vi "Main Page.vi"(8 "error in (no error)":errorcluster, 11 "Node Ptr":T1 format="%.0x") -> (0 "error out":errorcluster)   [LabVIEW 2024, in "Nominal Client System Explorer.lvlib"]
uses:
  Nominal Client System Explorer.lvlib
  <vilib>/NI VeriStand/Custom Device API/Custom Device Item Ref.ctl
  <vilib>/NI VeriStand/Custom Device API/Get Item Property (U16).vi
  <vilib>/NI VeriStand/Custom Device API/Set Item Property (U16).vi
  <vilib>/NI VeriStand/Custom Device API/Custom Device API.lvlib
  Scripting/Nominal Client Scripting.lvlib
  <vilib>/NI VeriStand/Custom Device Tools/Custom Device Utility Library/Custom Device Utility Library.lvlib
panel:
  in  "Remove":bool
  in  "Channels to Stream":i32[](listbox)
  in  "Add Channels":bool
  in  "Datasource Connection Name":string
  in  "Path to API Token file":path caption="A text file containing your API Token only."
  in  "Description":string
  in  "Name":string
  out "Version":string
  in  "General Header":cluster{"Section Name":string}={"Section Name"="Nominal IO VeriStand Client Details"}
  in  "Specific Header":cluster{"Section Name":string}={"Section Name"="Settings"}
  in  "Async Timeout (ms)":u16
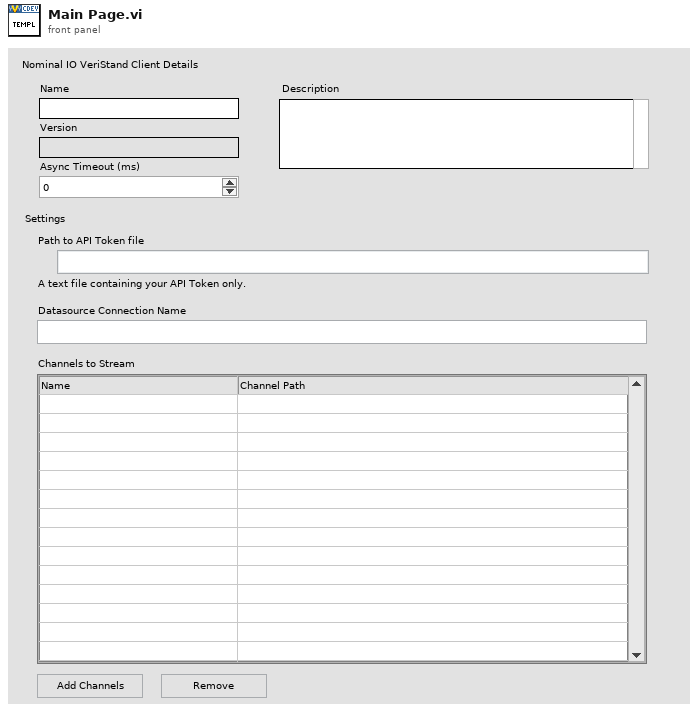
[diagram p1: front panel]
types:
  T1 = typedef "Custom Device API.lvlib/Custom Device Item Ref.ctl" = u64
  T2 = typedef "Custom Device API.lvlib/Custom Device Item Info.ctl" = cluster{"Name":string, "Is Channel":bool, "GUID":string, "Is Waveform":bool}
  T3 = typedef "Custom Device API.lvlib/Custom Device Commands.ctl" = enum16{"Default", "Item renamed", "Shutdown", "Dynamic button pressed"}
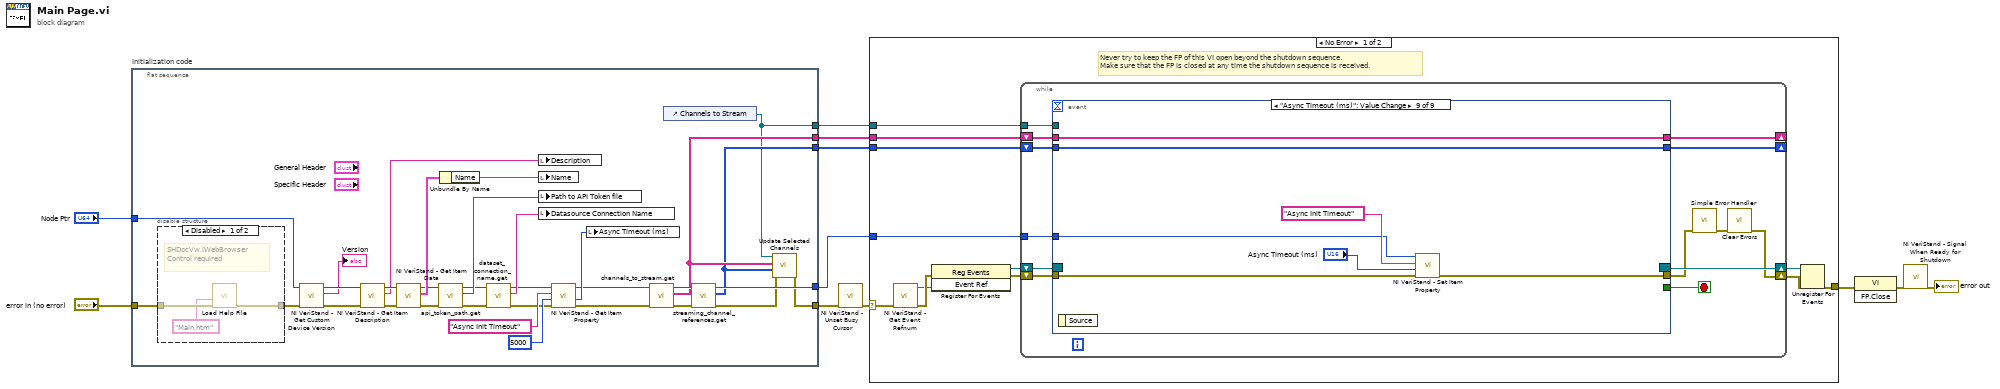
[diagram p0: block diagram]
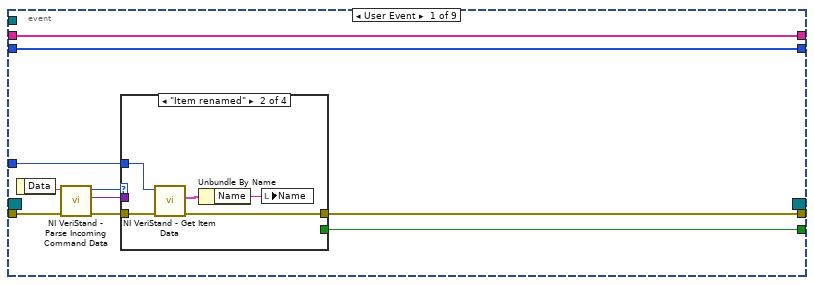
[diagram p2: hidden frame]
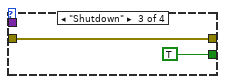
[diagram p4: hidden frame]
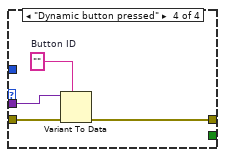
[diagram p5: hidden frame]
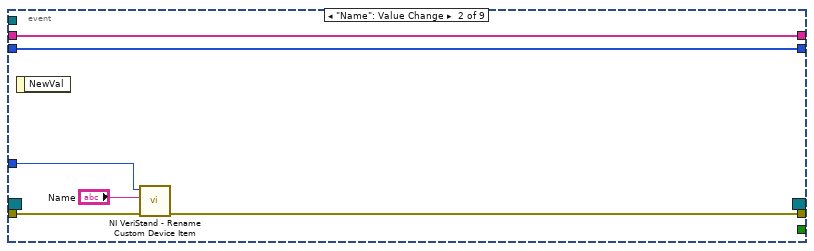
[diagram p6: hidden frame]
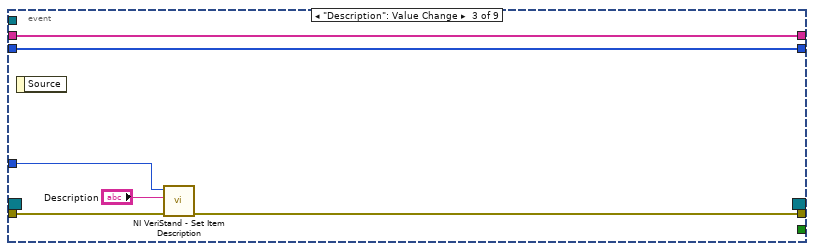
[diagram p7: hidden frame]
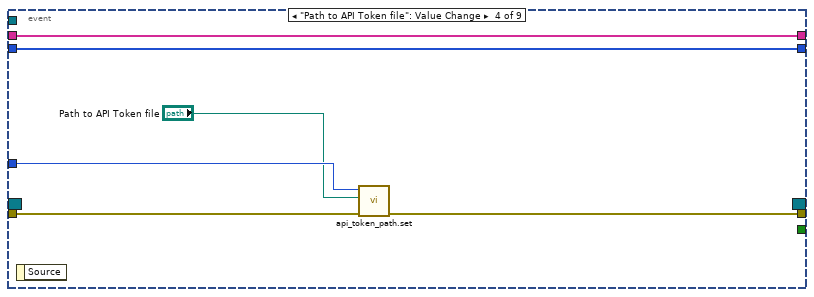
[diagram p8: hidden frame]
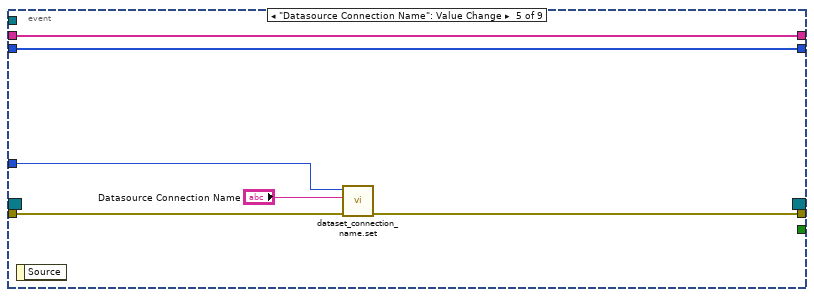
[diagram p9: hidden frame]
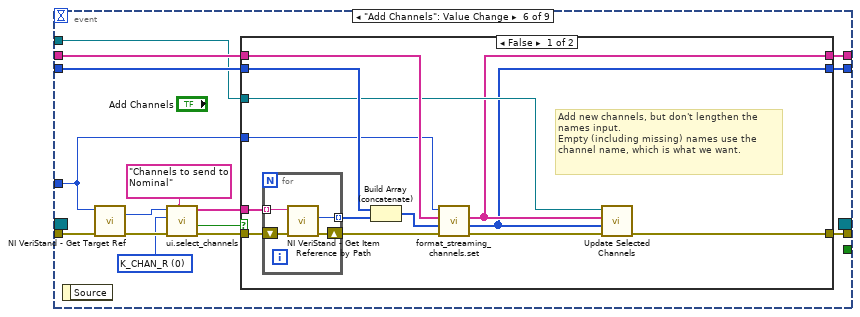
[diagram p10: hidden frame]
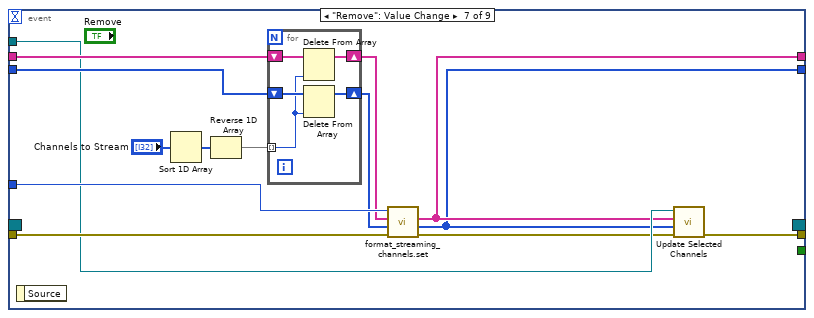
[diagram p12: hidden frame]
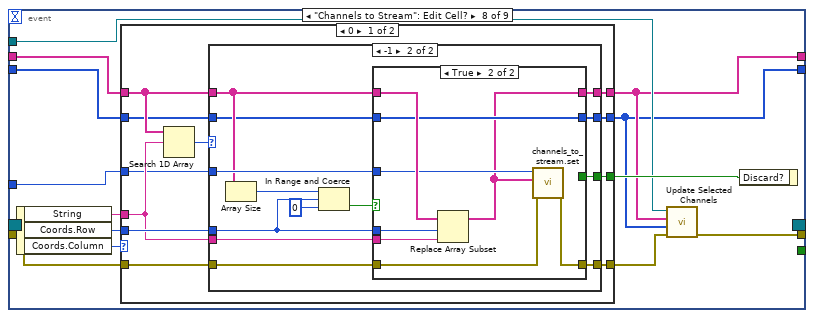
[diagram p13: hidden frame]
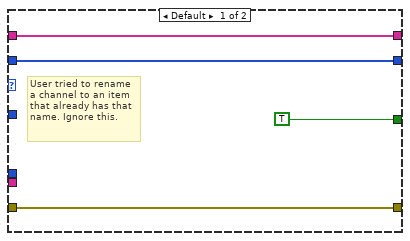
[diagram p14: hidden frame]
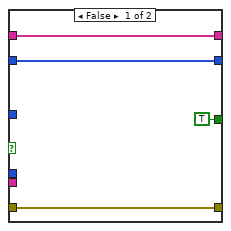
[diagram p15: hidden frame]
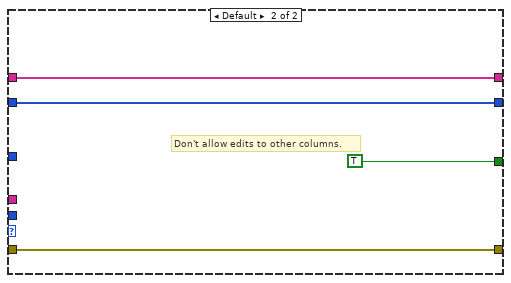
[diagram p16: hidden frame]
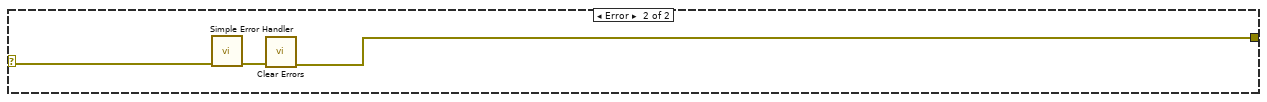
[diagram p17: hidden frame]
diagram:
  n1 = flat-sequence "Initialization code" {
    tunnel: "error in (no error)" -> [w34]
    tunnel: "Node Ptr" -> [w40]
    tunnel: [w20] -> w8
    tunnel: [w26] -> w6
    tunnel: [w22] -> w5
    tunnel: [w23] -> w4
    tunnel: [w19] -> w3
    frame #0 {
      n2 = disable-structure shown="Disabled" {
        disable-tunnel: w34 -> [w46 w47]
        disable-tunnel: [w44 w47] -> w33
        frame Disabled {
          # "SHDocVw.IWebBrowser Control required"
          n3 = call "Load Help File.vi"("error in (no error)"=w46, "HTML File to Load"="Main.htm" ("HTML File")) -> ("error out"=w44:errorcluster)  [unwired: 9 in]
        }
        frame Enabled {
          # "Enable to add help support"
        }
      }
      n4 = call <vilib>:"NI VeriStand - Get Custom Device Version.vi"("error in (no error)"=w33, "Device Ref in"=w40) -> ("error out"=w39:errorcluster, "Value"=→"Version":string, "Device Ref out"=w38:T1)  [unwired: 7 in]
      n5 = call <vilib>:"NI VeriStand - Get Item Description.vi"("error in (no error)"=w39, "Item Ref in"=w38) -> ("error out"=w42:errorcluster, "Description"=w35:string, "Item Ref out"=w43:T1)  [unwired: 7 out]
      n6 = call <vilib>:"NI VeriStand - Get Item Data.vi"("error in (no error)"=w42, "Item Ref in"=w43) -> ("error out"=w31:errorcluster, "Item Info"=w41:T2, "Item Ref out"=w32:T1)  [unwired: 7 out]
      n7 = call "api_token_path.get.vi"("error in (no error)"=w31, "Nominal IO Client in"=w32) -> ("error out"=w28:errorcluster, "API Token file"=w30:path, "Nominal IO Client out"=w29:T1)  [unwired: 6 in, 1 out]
      n8 = Unbundle By Name(w41) -> ("Name"=w36:string)
      n9 = call "dataset_connection_name.get.vi"("error in (no error)"=w28, "Nominal IO Client in"=w29) -> ("error out"=w14:errorcluster, "dataset connection name"=w27:string, "Nominal IO Client out"=w15:T1)  [unwired: 6 in, 1 out]
      n10 = local write "Description"(w35) -> ()
      n11 = local write "Name"(w36) -> ()
      n12 = local write "Path to API Token file"(w30) -> ()
      n13 = local write "Datasource Connection Name"(w27) -> ()
      n14 = call-poly <vilib>:"NI VeriStand - Get Item Property.vi"("error in (no error)"=w14, "Default Value"=u16 5000, "Property Name"="Async Init Timeout", "Item Ref in"=w15) -> ("error out"=w13:errorcluster, "Value"=w18:u16, "Item Ref out"=w12:T1)  [unwired: 4 in, 1 out]
      n15 = local write "Async Timeout (ms)"(w18) -> ()
      n16 = call "channels_to_stream.get.vi"("error in (no error)"=w13, "Nominal IO Client in"=w12) -> ("error out"=w25:errorcluster, "Channels to Stream"=w23:string[], "Nominal IO Client out"=w24:T1)  [unwired: 6 in, 1 out]
      n17 = control-ref of="Channels to Stream"() -> (w19:refnum<vi>)
      n18 = call "streaming_channel_references.get.vi"("error in (no error)"=w25, "Item Ref in"=w24) -> ("error out"=w21:errorcluster, "Streaming Channel Refs"=w22:T1[], "Item Ref out"=w26:T1)  [unwired: 7 in]
      n19 = call "Update Selected Channels.vi"("error in"=w21, "Channel Refs"=w22, "Channel Names"=w23, "Listbox"=w19) -> ("error out"=w20:errorcluster)  [unwired: 7 in]
    }
  }
  n20 = call <vilib>:"NI VeriStand - Unset Busy Cursor.vi"("error in (no error)"=w8) -> ("error out"=w7:errorcluster)  [unwired: 10 out]
  n21 = case shown="No Error" w7 {
    selector: w7 -> [w51 w239]
    tunnel: [w56 w237] -> w11
    tunnel: w6 -> [w52 _]
    tunnel: w5 -> [w50 _]
    tunnel: w4 -> [w49 _]
    tunnel: w3 -> [w48 _]
    frame No Error {
      # "Never try to keep the FP of this VI open beyond the shutdown sequence.\nMake sure that the FP is closed at any time the shutdown sequence is received."
      n22 = call <vilib>:"NI VeriStand - Get Event Refnum.vi"("error in (no error)"=w51) -> ("error out"=w59:errorcluster, "Event Ref"=w55:refnum<user-event>)  [unwired: 9 out]
      n23 = register-events(error in=w59, w55) -> (reference out=w53:refnum<event-registration>, error out=w54:errorcluster)  [unwired: 1 in]
      n24 = while {
        tunnel: w52 -> [w68]
        shift-right: [w65] -> w57
        shift-left: w54 -> [w71]
        shift-right: [w72] -> w58
        shift-left: w53 -> [w70]
        shift-right: [w63] -> _
        shift-left: w50 -> [w64]
        shift-right: [w61] -> _
        shift-left: w49 -> [w62]
        tunnel: w48 -> [w60]
        stop <- w69 stop-if-true
        n25 = event shown="[8] \"Async Timeout (ms)\": Value Change" {
          selector: w70 -> [_ _ _ _ _ _ _ _ _]
          dyn-events: [_ _ _ _ _ _ _ _ _] -> w72
          timeout: _ -> [_ _ _ _ _ _ _ _ _]
          tunnel: w71 -> [w82 w100 w105 w110 w115 w133 w159 w182 w231]
          tunnel: [w73 _ _ _ _ _ _ _ _] -> w69
          tunnel: [w74 w99 w104 w109 w116 w128 w154 w173 w230] -> w67
          tunnel: w68 -> [w75 w98 w106 w112 w117 w127 w162 w183 w232]
          tunnel: w64 -> [w76 w95 w101 w107 w113 w132 w165 w185 w236]
          tunnel: [w76 w95 w101 w107 w113 w131 w156 w175 w236] -> w63
          tunnel: w62 -> [w77 w96 w102 w108 w114 w130 w164 w184 w235]
          tunnel: [w77 w96 w102 w108 w114 w129 w157 w176 w235] -> w61
          tunnel: w60 -> [_ _ _ _ _ w126 w158 w177 _]
          event User Event {
            n26 = event-data() -> ("Data"=w81:string)  [unwired: 1 out]
            n27 = call <vilib>:"NI VeriStand - Parse Incoming Command Data.vi"("error in (no error)"=w82, "Incoming data"=w81) -> ("error out"=w80:errorcluster, "Outgoing data"=w78:variant, "Action"=w79:T3)  [unwired: 7 out]
            n28 = case shown="\"Item renamed\"" w79 {
              tunnel: w80 -> [w83 w88 w89 w94]
              tunnel: [_ _ TRUE _] -> w73
              tunnel: [w83 w85 w89 w91] -> w74
              tunnel: w75 -> [_ w87 _ _]
              tunnel: w78 -> [_ _ _ w93]
              frame "Default", Default {
              }
              frame "Item renamed" {
                n29 = call <vilib>:"NI VeriStand - Get Item Data.vi"("error in (no error)"=w88, "Item Ref in"=w87) -> ("error out"=w85:errorcluster, "Item Info"=w86:T2)  [unwired: 8 out]
                n30 = Unbundle By Name(w86) -> ("Name"=w84:string)
                n31 = local write "Name"(w84) -> ()
              }
              frame "Shutdown" {
              }
              frame "Dynamic button pressed" {
                w92 = ""  # Button ID
                n32 = Variant To Data(error in=w94, type=w92, Variant=w93) -> (error out=w91:errorcluster)  [unwired: 1 out]
              }
            }
          }
          event "Name": Value Change {
            n33 = event-data() -> ()  [unwired: 2 out]
            n34 = call <vilib>:"NI VeriStand - Rename Custom Device Item.vi"("error in (no error)"=w100, "New Name"="Name", "Item Ref in"=w98) -> ("error out"=w99:errorcluster)  [unwired: 1 in, 7 out]
          }
          event "Description": Value Change {
            n35 = event-data() -> ()  [unwired: 2 out]
            n36 = call <vilib>:"NI VeriStand - Set Item Description.vi"("error in (no error)"=w105, "Description"="Description", "Item Ref in"=w106) -> ("error out"=w104:errorcluster)  [unwired: 8 out]
          }
          event "Path to API Token file": Value Change {
            n37 = event-data() -> ()  [unwired: 2 out]
            n38 = call "api_token_path.set.vi"("error in (no error)"=w110, "API Token file"="Path to API Token file", "Nominal IO Client in"=w112) -> ("error out"=w109:errorcluster)  [unwired: 6 in, 2 out]
          }
          event "Datasource Connection Name": Value Change {
            n39 = event-data() -> ()  [unwired: 2 out]
            n40 = call "dataset_connection_name.set.vi"("error in (no error)"=w115, "dataset connection name"="Datasource Connection Name", "Nominal IO Client in"=w117) -> ("error out"=w116:errorcluster)  [unwired: 6 in, 2 out]
          }
          event "Add Channels": Value Change {
            w119 = u8 0 items=["K_CHAN_R", "K_CHAN_W", "K_CHAN_RW", "K_CHAN_VOLT", "K_CHAN_FAULT", "K_ALL", "K_CUSTOM"] ("Filter")
            n41 = event-data() -> ()  [unwired: 2 out]
            n42 = call <vilib>:"NI VeriStand - Get Target Ref.vi"("error in"=w133, "Item Ref in"=w127) -> ("error out"=w124:errorcluster, "Target Ref"=w123:T1)  [unwired: 6 in, 2 out]
            n43 = call "ui.select_channels.vi"("Channel Label"="Channels to send to Nominal", "error in (no error)"=w124, "Filter"=w119, "Start Item Ref"=w123) -> ("error out"=w122:errorcluster, "Canceled"=w121:bool, "Channels"=w120:string[])  [unwired: 5 in]
            n44 = case shown="False" w121 {
              tunnel: w120 -> [w146 _]
              tunnel: w122 -> [w145 w151]
              tunnel: w132 -> [w142 w152]
              tunnel: [w136 w152] -> w131
              tunnel: w130 -> [w141 w153]
              tunnel: [w137 w153] -> w129
              tunnel: [w134 w151] -> w128
              tunnel: w127 -> [w139 _]
              tunnel: w126 -> [w138 _]
              frame False {
                # "Add new channels, but don't lengthen the names input.\nEmpty (including missing) names use the channel name, which is what we want."
                n45 = for {
                  shift-right: [w149] -> w140
                  shift-left: w145 -> [w150]
                  tunnel: w146 -> [w148] mode=indexing
                  tunnel: [w147] -> w144 mode=indexing
                  n46 = call <vilib>:"NI VeriStand - Get Item Reference by Path.vi"("error in (no error)"=w150, "Item Path in"=w148) -> ("error out"=w149:errorcluster, "Item Ref"=w147:T1)  [unwired: 6 in, 2 out]
                }
                n47 = Build Array (concatenate)(w142, w144) -> (w143:T1[])
                n48 = call "format_streaming_channels.set.vi"("error in"=w140, "channels"=w143, "names"=w141, "Nominal IO Client in"=w139) -> ("error out"=w135:errorcluster, "saved channels"=w136:T1[], "saved names"=w137:string[])  [unwired: 4 in, 1 out]
                n49 = call "Update Selected Channels.vi"("error in"=w135, "Channel Refs"=w136, "Channel Names"=w137, "Listbox"=w138) -> ("error out"=w134:errorcluster)  [unwired: 7 in]
              }
              frame True {
              }
            }
          }
          event "Remove": Value Change {
            n50 = event-data() -> ()  [unwired: 2 out]
            n51 = Sort 1D Array(array="Channels to Stream") -> (sorted array=w167:i32[])
            n52 = Reverse 1D Array(array=w167) -> (reversed array=w166:i32[])
            n53 = for {
              shift-right: [w171] -> w160
              shift-left: w165 -> [w172]
              tunnel: w166 -> [w168] mode=indexing
              shift-right: [w169] -> w161
              shift-left: w164 -> [w170]
              n54 = Delete From Array(array=w170, index=w168) -> (array with subset deleted=w169:string[])  [unwired: 1 in, 1 out]
              n55 = Delete From Array(array=w172, index=w168) -> (array with subset deleted=w171:T1[])  [unwired: 1 in, 1 out]
            }
            n56 = call "format_streaming_channels.set.vi"("error in"=w159, "channels"=w160, "names"=w161, "Nominal IO Client in"=w162) -> ("error out"=w155:errorcluster, "saved channels"=w156:T1[], "saved names"=w157:string[])  [unwired: 4 in, 1 out]
            n57 = call "Update Selected Channels.vi"("error in"=w155, "Channel Refs"=w156, "Channel Names"=w157, "Listbox"=w158) -> ("error out"=w154:errorcluster)  [unwired: 7 in]
          }
          event "Channels to Stream": Edit Cell? {
            n58 = event-data() -> ("String"=w178:string, "Coords.Row"=w179:i32, "Coords.Column"=w181:i32)  [unwired: 1 out]
            n59 = case shown="0" w181 {
              tunnel: w185 -> [w191 w228]
              tunnel: w184 -> [w193 w229]
              tunnel: [w194 w229] -> w176
              tunnel: [w192 w228] -> w175
              tunnel: w179 -> [w190 _]
              tunnel: [w195 TRUE] -> w180
              tunnel: w178 -> [w189 _]
              tunnel: w182 -> [w188 w226]
              tunnel: w183 -> [w187 _]
              tunnel: [w186 w226] -> w174
              frame 0 {
                n60 = Search 1D Array(1D array=w193, element=w189) -> (index of element=w196:i32)  [unwired: 1 in]
                n61 = case shown="-1" w196 {
                  tunnel: [TRUE w201] -> w195
                  tunnel: [w199 w210] -> w194
                  tunnel: w193 -> [w199 w208]
                  tunnel: [w198 w207] -> w192
                  tunnel: w191 -> [w198 w206]
                  tunnel: w190 -> [_ w204]
                  tunnel: w189 -> [_ w213]
                  tunnel: w188 -> [w197 w212]
                  tunnel: w187 -> [_ w211]
                  tunnel: [w197 w209] -> w186
                  frame Default {
                    # "User tried to rename a channel to an item that already has that name. Ignore this."
                  }
                  frame -1 {
                    n62 = Array Size(array=w208) -> (size(s)=w205:i32)
                    n63 = In Range and Coerce(upper limit=w205, x=w204, lower limit=0) -> (In Range?=w203:bool)  [unwired: 1 out]
                    n64 = case shown="True" w203 {
                      tunnel: w204 -> [_ w225]
                      tunnel: w213 -> [_ w224]
                      tunnel: w212 -> [w215 w219]
                      tunnel: w211 -> [_ w221]
                      tunnel: [w217 w220] -> w210
                      tunnel: [w215 w218] -> w209
                      tunnel: w208 -> [w217 w223]
                      tunnel: [w216 w222] -> w207
                      tunnel: w206 -> [w216 w222]
                      tunnel: [TRUE _] -> w201
                      frame False {
                      }
                      frame True {
                        n65 = Replace Array Subset(array=w223, new element=w224, index=w225) -> (w220:string[])
                        n66 = call "channels_to_stream.set.vi"("error in (no error)"=w219, "Channels to Stream"=w220, "Nominal IO Client in"=w221) -> ("error out"=w218:errorcluster)  [unwired: 6 in, 2 out]
                      }
                    }
                  }
                }
              }
              frame Default {
                # "Don't allow edits to other columns."
              }
            }
            n67 = call "Update Selected Channels.vi"("error in"=w174, "Channel Refs"=w175, "Channel Names"=w176, "Listbox"=w177) -> ("error out"=w173:errorcluster)  [unwired: 7 in]
            n68 = event-data("Discard?"=w180) -> ()  [unwired: 1 in, 1 out]
          }
          event "Async Timeout (ms)": Value Change {
            n69 = event-data() -> ()  [unwired: 2 out]
            n70 = call-poly <vilib>:"NI VeriStand - Set Item Property.vi"("error in (no error)"=w231, "Value"="Async Timeout (ms)", "Property Name"="Async Init Timeout", "Item Ref in"=w232) -> ("error out"=w230:errorcluster)  [unwired: 5 in, 2 out]
          }
        }
        n71 = call <vilib>:"Simple Error Handler.vi"("error in (no error)"=w67) -> ("error out"=w66:errorcluster)  [unwired: 1 in, 7 out]
        n72 = call <vilib>:"Clear Errors.vi"("error in (no error)"=w66) -> ("error out"=w65:errorcluster)  [unwired: 1 in, 5 out]
      }
      n73 = Unregister For Events(event registration refnum=w58, error in=w57) -> (error out=w56:errorcluster)
    }
    frame Error {
      n74 = call <vilib>:"Simple Error Handler.vi"("error in (no error)"=w239) -> ("error out"=w238:errorcluster)  [unwired: 1 in, 7 out]
      n75 = call <vilib>:"Clear Errors.vi"("error in (no error)"=w238) -> ("error out"=w237:errorcluster)  [unwired: 1 in, 5 out]
    }
  }
  n76 = invoke class="VI" method="FP.Close"(error in=w11) -> (error out=w10:errorcluster)  [unwired: 2 in, 2 out]
  n77 = call <vilib>:"NI VeriStand - Signal When Ready for Shutdown.vi"("error in (no error)"=w10) -> ("error out"=→"error out":errorcluster)  [unwired: 10 out]
